vi "Translate Raw Sample Data.vi"(8 "Error In":errorcluster, 10 "Sample Raw Data":T4, 11 "Open Weather Session In":refnum<class "Open Weather Session.lvclass">) -> (0 "Error Out":errorcluster, 2 "Weather Sample Data":T1, 3 "Open Weather Session Out":refnum<class "Open Weather Session.lvclass">)   [LabVIEW 2019, in "Open Weather Session.lvclass"]
uses:
  Open Weather Session.lvclass
  Controls/Weather Sample Raw Data.ctl
  Controls/Weather Description Raw Data.ctl
  Public/Controls/Weather Sample Data.ctl
  <vilib>/Utility/miscctls.llb/LVDateTimeRec.ctl
  Public/Controls/Weather Description Data.ctl
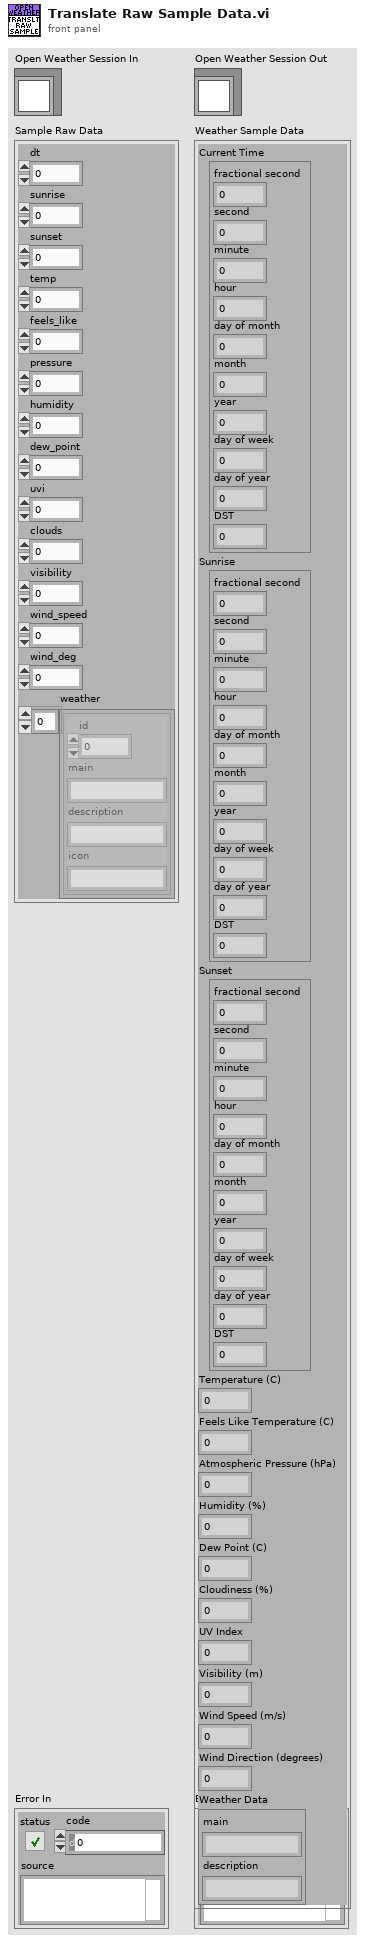
[diagram p1: front panel]
types:
  T1 = typedef "Open Weather Session.lvclass/Weather Sample Data.ctl" = cluster{"Current Time":T2, "Sunrise":T2, "Sunset":T2, "Temperature (C)":dbl, "Feels Like Temperature (C)":dbl, "Atmospheric Pressure (hPa)":dbl, "Humidity (%)":dbl, "Dew Point (C)":dbl, "Cloudiness (%)":dbl, "UV Index":dbl, "Visibility (m)":dbl, "Wind Speed (m/s)":dbl, "Wind Direction (degrees)":dbl, "Weather Data":T3}
  T2 = typedef "LVDateTimeRec.ctl" = cluster{"fractional second":dbl, "second":i32, "minute":i32, "hour":i32, "day of month":i32, "month":i32, "year":i32, "day of week":i32, "day of year":i32, "DST":i32}
  T3 = typedef "Open Weather Session.lvclass/Weather Description Data.ctl" = cluster{"main":string, "description":string}
  T4 = typedef "Open Weather Session.lvclass/Weather Sample Raw Data.ctl" = cluster{"dt":dbl, "sunrise":dbl, "sunset":dbl, "temp":dbl, "feels_like":dbl, "pressure":i32, "humidity":i32, "dew_point":dbl, "uvi":dbl, "clouds":i32, "visibility":i32, "wind_speed":dbl, "wind_deg":i32, "weather":T5[]}
  T5 = typedef "Open Weather Session.lvclass/Weather Description Raw Data.ctl" = cluster{"id":u32, "main":string, "description":string, "icon":string}
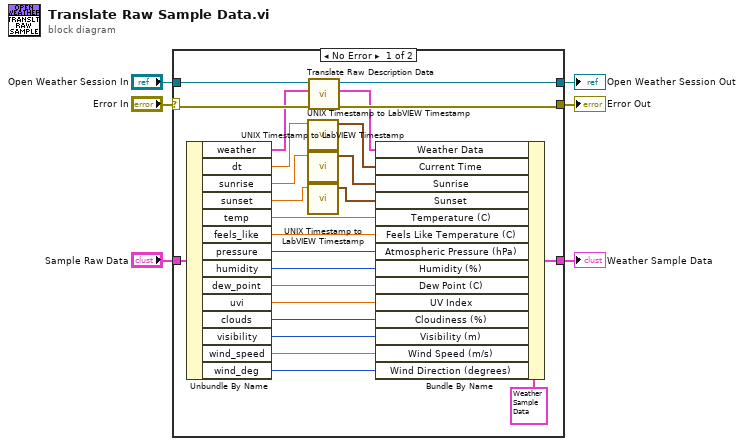
[diagram p0: block diagram]
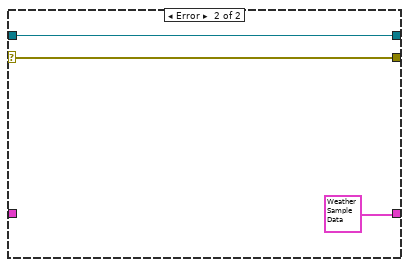
[diagram p2: hidden frame]
diagram:
  n1 = case shown="No Error" "Error In" {
    selector: "Error In" -> [w18 w33]
    tunnel: [w16 w34] -> w6
    tunnel: [w14 w33] -> w5
    tunnel: "Open Weather Session In" -> [w17 w34]
    tunnel: "Sample Raw Data" -> [w31 _]
    tunnel: [w19 T1 {"Current Time"={"fractional second"=0.0, "second"=0, "minute"=0, "hour"=0, "day of month"=0, "month"=0, "year"=0, "day of week"=0, "day of year"=0, "DST"=0}, "Sunrise"={"fractional second"=0.0, "second"=0, "minute"=0, "hour"=0, "day of month"=0, "month"=0, "year"=0, "day of week"=0, "day of year"=0, "DST"=0}, "Sunset"={"fractional second"=0.0, "second"=0, "minute"=0, "hour"=0, "day of month"=0, "month"=0, "year"=0, "day of week"=0, "day of year"=0, "DST"=0}, "Temperature (C)"=0.0, "Feels Like Temperature (C)"=0.0, "Atmospheric Pressure (hPa)"=0.0, "Humidity (%)"=0.0, "Dew Point (C)"=0.0, "Cloudiness (%)"=0.0, "UV Index"=0.0, "Visibility (m)"=0.0, "Wind Speed (m/s)"=0.0, "Wind Direction (degrees)"=0.0, "Weather Data"={"main"="", "description"=""}} ("Weather Sample Data")] -> w1
    frame No Error {
      n2 = Unbundle By Name(w31) -> ("weather"=w15:T5[], "dt"=w12:dbl, "sunrise"=w8:dbl, "sunset"=w10:dbl, "temp"=w29:dbl, "feels_like"=w28:dbl, "pressure"=w27:i32, "humidity"=w26:i32, "dew_point"=w25:dbl, "uvi"=w24:dbl, "clouds"=w23:i32, "visibility"=w22:i32, "wind_speed"=w21:dbl, "wind_deg"=w20:i32)
      n3 = call "UNIX Timestamp to LabVIEW Timestamp.vi"("UNIX time stamp"=w12) -> ("LabVIEW Timestamp"=w11:T2)  [unwired: 10 in]
      n4 = call "UNIX Timestamp to LabVIEW Timestamp.vi"("UNIX time stamp"=w8) -> ("LabVIEW Timestamp"=w7:T2)  [unwired: 10 in]
      n5 = call "UNIX Timestamp to LabVIEW Timestamp.vi"("UNIX time stamp"=w10) -> ("LabVIEW Timestamp"=w9:T2)  [unwired: 10 in]
      n6 = call "Translate Raw Description Data.vi"("Error In"=w18, "Weather Description Raw Data"=w15, "Open Weather Session In"=w17) -> ("Error Out"=w14:errorcluster, "Weather Data"=w13:T3, "Open Weather Session Out"=w16:refnum<class "Open Weather Session.lvclass">)  [unwired: 6 in]
      n7 = Bundle By Name(cluster=T1 {"Current Time"={"fractional second"=0.0, "second"=0, "minute"=0, "hour"=0, "day of month"=0, "month"=0, "year"=0, "day of week"=0, "day of year"=0, "DST"=0}, "Sunrise"={"fractional second"=0.0, "second"=0, "minute"=0, "hour"=0, "day of month"=0, "month"=0, "year"=0, "day of week"=0, "day of year"=0, "DST"=0}, "Sunset"={"fractional second"=0.0, "second"=0, "minute"=0, "hour"=0, "day of month"=0, "month"=0, "year"=0, "day of week"=0, "day of year"=0, "DST"=0}, "Temperature (C)"=0.0, "Feels Like Temperature (C)"=0.0, "Atmospheric Pressure (hPa)"=0.0, "Humidity (%)"=0.0, "Dew Point (C)"=0.0, "Cloudiness (%)"=0.0, "UV Index"=0.0, "Visibility (m)"=0.0, "Wind Speed (m/s)"=0.0, "Wind Direction (degrees)"=0.0, "Weather Data"={"main"="", "description"=""}} ("Weather Sample Data"), "Weather Data"=w13, "Current Time"=w11, "Sunrise"=w7, "Sunset"=w9, "Temperature (C)"=w29, "Feels Like Temperature (C)"=w28, "Atmospheric Pressure (hPa)"=w27, "Humidity (%)"=w26, "Dew Point (C)"=w25, "UV Index"=w24, "Cloudiness (%)"=w23, "Visibility (m)"=w22, "Wind Speed (m/s)"=w21, "Wind Direction (degrees)"=w20) -> (w19:T1)
    }
    frame Error {
    }
  }
  "Open Weather Session Out" <- w6
  "Error Out" <- w5
  "Weather Sample Data" <- w1
